vi "GetGenealogyItemData.vi"(1 "Genealogy Item":T2) -> (0 "GenealogyItemData":T1 {"ID" format="%x"})   [LabVIEW 2021, in "Lunar UDS CAN.lvlib"]
doc: "Defines the genealogy item data for each genealogy item."
uses:
  Lunar UDS CAN.lvlib
  Controls/UDSGenealogyItems.ctl
  Controls/UDSGenealoogyItemData.ctl
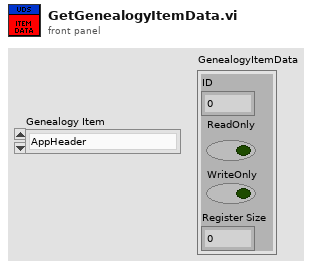
[diagram p1: front panel]
types:
  T1 = typedef "Lunar UDS CAN.lvlib/UDSGenealoogyItemData.ctl" = cluster{"ID":i32, "ReadOnly":bool, "WriteOnly":bool, "Register Size":i32}
  T2 = typedef "Lunar UDS CAN.lvlib/UDSGenealogyItems.ctl" = enum16{"AppHeader", "Genealogy Block Init", "Genealogy Block", "Board Part Number", "Board Serial Number", "Aux1 Part Number", "Aux1 Serial Number", "Aux2 Part Number", "Aux2 Serial Number", "Config Block Init", "Config Block", "Calibration Block Init", "Calibration Block", "Node Data Block Init", "Node Data Block", "Can Bus Instance"}
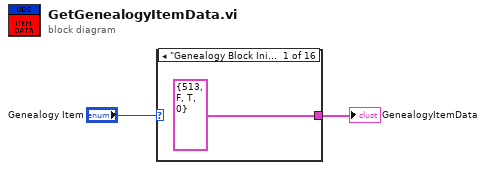
[diagram p0: block diagram]
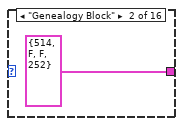
[diagram p2: hidden frame]
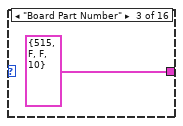
[diagram p3: hidden frame]
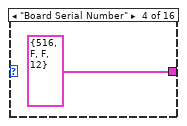
[diagram p4: hidden frame]
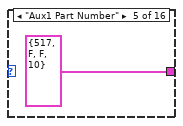
[diagram p5: hidden frame]
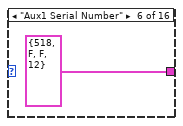
[diagram p6: hidden frame]
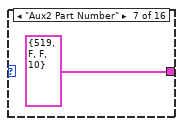
[diagram p7: hidden frame]
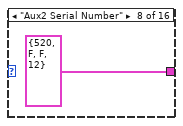
[diagram p8: hidden frame]
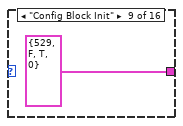
[diagram p9: hidden frame]
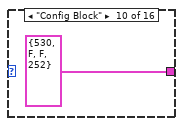
[diagram p10: hidden frame]
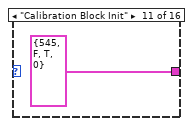
[diagram p11: hidden frame]
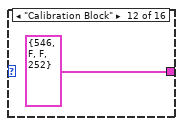
[diagram p12: hidden frame]
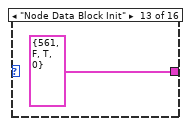
[diagram p13: hidden frame]
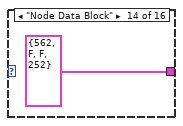
[diagram p14: hidden frame]
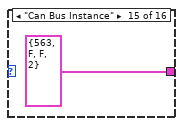
[diagram p15: hidden frame]
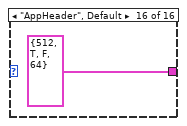
[diagram p16: hidden frame]
diagram:
  n1 = case shown="\"Genealogy Block Init\"" "Genealogy Item" {
    tunnel: [T1 {"ID"=513, "ReadOnly"=FALSE, "WriteOnly"=TRUE, "Register Size"=0} ("GenealogyItemData") T1 {"ID"=514, "ReadOnly"=FALSE, "WriteOnly"=FALSE, "Register Size"=252} ("GenealogyItemData") T1 {"ID"=515, "ReadOnly"=FALSE, "WriteOnly"=FALSE, "Register Size"=10} ("GenealogyItemData") T1 {"ID"=516, "ReadOnly"=FALSE, "WriteOnly"=FALSE, "Register Size"=12} ("GenealogyItemData") T1 {"ID"=517, "ReadOnly"=FALSE, "WriteOnly"=FALSE, "Register Size"=10} ("GenealogyItemData") T1 {"ID"=518, "ReadOnly"=FALSE, "WriteOnly"=FALSE, "Register Size"=12} ("GenealogyItemData") T1 {"ID"=519, "ReadOnly"=FALSE, "WriteOnly"=FALSE, "Register Size"=10} ("GenealogyItemData") T1 {"ID"=520, "ReadOnly"=FALSE, "WriteOnly"=FALSE, "Register Size"=12} ("GenealogyItemData") T1 {"ID"=529, "ReadOnly"=FALSE, "WriteOnly"=TRUE, "Register Size"=0} ("GenealogyItemData") T1 {"ID"=530, "ReadOnly"=FALSE, "WriteOnly"=FALSE, "Register Size"=252} ("GenealogyItemData") T1 {"ID"=545, "ReadOnly"=FALSE, "WriteOnly"=TRUE, "Register Size"=0} ("GenealogyItemData") T1 {"ID"=546, "ReadOnly"=FALSE, "WriteOnly"=FALSE, "Register Size"=252} ("GenealogyItemData") T1 {"ID"=561, "ReadOnly"=FALSE, "WriteOnly"=TRUE, "Register Size"=0} ("GenealogyItemData") T1 {"ID"=562, "ReadOnly"=FALSE, "WriteOnly"=FALSE, "Register Size"=252} ("GenealogyItemData") T1 {"ID"=563, "ReadOnly"=FALSE, "WriteOnly"=FALSE, "Register Size"=2} ("GenealogyItemData") T1 {"ID"=512, "ReadOnly"=TRUE, "WriteOnly"=FALSE, "Register Size"=64} ("GenealogyItemData")] -> w1
    frame "Genealogy Block Init" {
    }
    frame "Genealogy Block" {
    }
    frame "Board Part Number" {
    }
    frame "Board Serial Number" {
    }
    frame "Aux1 Part Number" {
    }
    frame "Aux1 Serial Number" {
    }
    frame "Aux2 Part Number" {
    }
    frame "Aux2 Serial Number" {
    }
    frame "Config Block Init" {
    }
    frame "Config Block" {
    }
    frame "Calibration Block Init" {
    }
    frame "Calibration Block" {
    }
    frame "Node Data Block Init" {
    }
    frame "Node Data Block" {
    }
    frame "Can Bus Instance" {
    }
    frame "AppHeader", Default {
    }
  }
  "GenealogyItemData" <- w1
